vi "Register Pin Map.vi"(8 "error in":errorcluster, 11 "pin map xml":string) -> (0 "error out":errorcluster, 3 "pin map id":string)   [LabVIEW 2020, in "MeasurementServerTests.lvlib"]
uses:
  MeasurementServerTests.lvlib
  Runtime/Generated/Measurement Plugin Pin Map Client/RPC Messages/ni_measurementlink_pinmap_v1_UpdatePinMapFromXmlRequest.ctl
  Runtime/Generated/Measurement Plugin Pin Map Client/Measurement Plugin Pin Map Client.lvlib
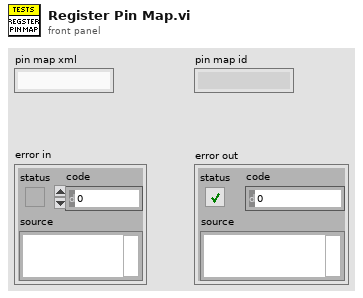
[diagram p1: front panel]
types:
  T1 = typedef "Measurement Plugin Pin Map Client.lvlib/ni_measurementlink_pinmap_v1_UpdatePinMapFromXmlRequest.ctl" = cluster{"pin_map_id":string, "pin_map_xml":string}
  T2 = typedef "Measurement Plugin Pin Map Client.lvlib/ni_measurementlink_pinmap_v1_PinMap.ctl" = cluster{"pin_map_id":string}
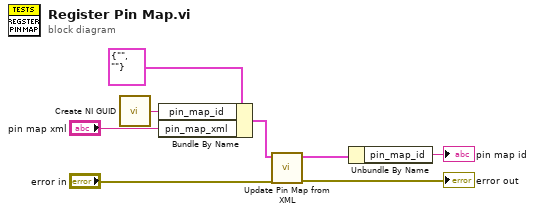
[diagram p0: block diagram]
diagram:
  n1 = call <vilib>:"Create NI GUID.vi"() -> ("NI GUID"=w7:string)
  n2 = Bundle By Name(cluster=T1 {"pin_map_id"="", "pin_map_xml"=""} ("Request Data"), "pin_map_id"=w7, "pin_map_xml"="pin map xml") -> (w1:T1)
  n3 = call "Update Pin Map from XML.vi"("error in"="error in", "request data"=w1) -> ("error out"=→"error out":errorcluster, "response data"=w2:T2)  [unwired: 8 in]
  n4 = Unbundle By Name(w2) -> ("pin_map_id"=→"pin map id":string)
